vi "VMCGUI.vi"(5 "error in (no error)":errorcluster) -> (16 "output cluster":T1, 19 "error out":errorcluster)   [LabVIEW 2018]
panel:
  in  "Mixer file (*.mxr)":path
  in  "Measurement":string(combo)="VC21"
  in  "Format":string(combo)="MLOGarithmic"
  in  "stop":bool
  in  "OK Button":bool
  # "VMC Measurement Parameters"
  # "The Mixer file must be stored locally on the PNA.\nMap to the PNA hard drive and select the Mixer\nfile to use for this measurement."
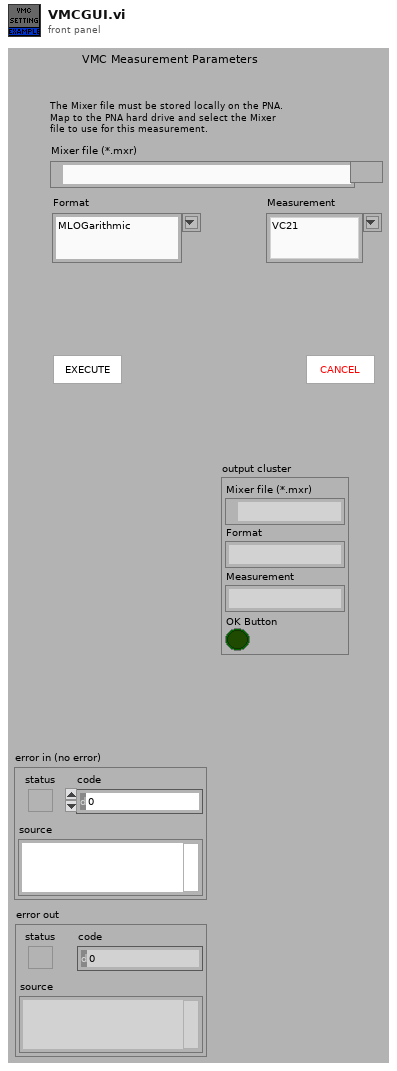
[diagram p1: front panel]
types:
  T1 = cluster{"Mixer file (*.mxr)":path, "Format":string, "Measurement":string, "OK Button":bool}
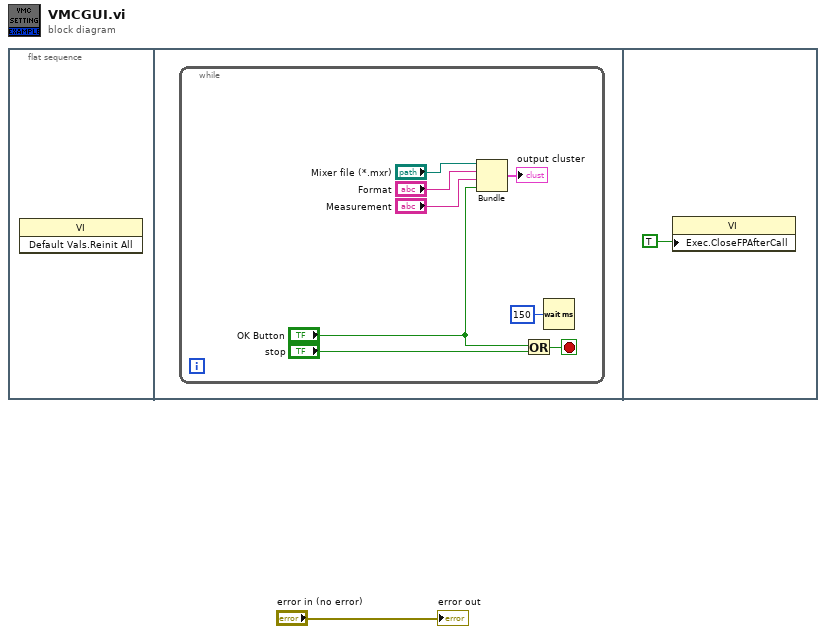
[diagram p0: block diagram]
diagram:
  n1 = flat-sequence {
    frame #0 {
      n2 = invoke class="VI" method="Default Vals.Reinit All"() -> ()  [unwired: 3 in, 3 out]
    }
    frame #1 {
      n3 = while {
        stop <- w8 stop-if-true
        n4 = Bundle("Mixer file (*.mxr)"="Mixer file (*.mxr)", "Format"="Format", "Measurement"="Measurement", "OK Button"="OK Button") -> (→"output cluster":T1)  [unwired: 1 in]
        n5 = Or(x="OK Button", y="stop") -> (x .or. y?=w8:bool)
        n6 = Wait (ms)(milliseconds to wait=u32 150) -> ()  [unwired: 1 out]
      }
    }
    frame #2 {
      n7 = property class="VI"("Exec.CloseFPAfterCall"=TRUE ("Execution:Close After Call")) -> ()  [unwired: 2 in, 2 out]
    }
  }
  "error out" <- "error in (no error)"
